vi "ppm wieder in Prozent umrechnen.vi"(6 "LNI_ppb":bool, 9 "Einheit":string, 11 "Werteingang":string) -> (3 "Wertausgang":string)   [LabVIEW 2020, in "Linearisierung v2.lvlib" / "Gasteiler.lvlib"]
uses:
  Gasteiler.lvlib
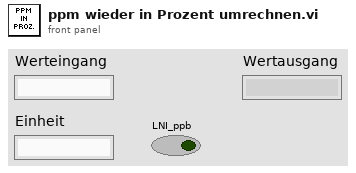
[diagram p1: front panel]
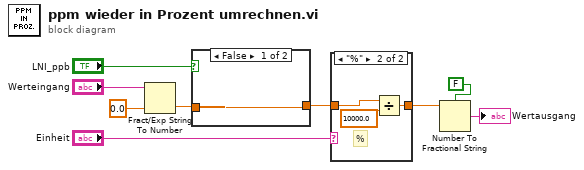
[diagram p0: block diagram]
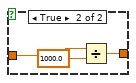
[diagram p2: hidden frame]
diagram:
  n1 = Fract/Exp String To Number(string="Werteingang", default (0 dbl)=sgl 0.0 ("x")) -> (number=w2:sgl)  [unwired: 2 in, 1 out]
  n2 = case shown="False" "LNI_ppb" {
    tunnel: w2 -> [w10 w13]
    tunnel: [w10 w11] -> w1
    frame False {
    }
    frame True {
      n3 = Divide(x=w13, y=sgl 1000.0) -> (x/y=w11:sgl)
    }
  }
  n4 = case shown="\"%\"" "Einheit" {
    tunnel: [w14 w16] -> w6
    tunnel: w1 -> [w14 w15]
    frame "ppm", Default {
      # "ppm"
    }
    frame "%" {
      # "%"
      n5 = Divide(x=w15, y=sgl 10000.0 ("x")) -> (x/y=w16:sgl)
    }
  }
  n6 = Number To Fractional String(use system decimal point (T)=FALSE ("Systemdezimalzeichen verwenden (T)"), number=w6) -> (F-format string=→"Wertausgang":string)  [unwired: 2 in]
